vi "ARM2 Reset parameters.vi"(0 "ARM2 Y-Galvo Offset":dbl, 1 "ARM2 Obejective Offset":dbl(slide) scale=0.0..10.0, 5 "ARM2 Z-Galvo Offset":dbl, 7 "ARM1 Z-Galvo Offset":dbl(slide) scale=0.0..10.0, 11 "ARM1 Obejective Offset":dbl(slide) scale=0.0..10.0, 12 "ARM1 Y-Galvo Offset":dbl(slide) scale=0.0..10.0) -> (4 "DAQ 2":waveform(dbl)[](array[waveform]), 15 "DAQ1":waveform(dbl)[](array[waveform]))   [LabVIEW 2016]
uses:
  <vilib>/measure/NI_MABase.lvlib
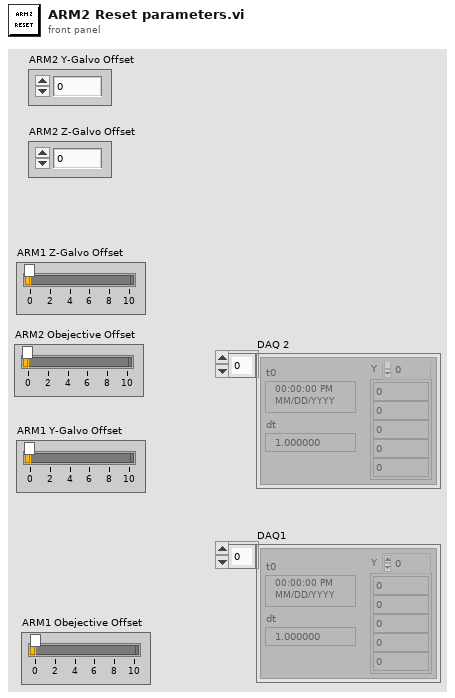
[diagram p1: front panel]
types:
  T1 = enum16{"Sine Wave", "Triangle Wave", "Square Wave", "Sawtooth Wave"}
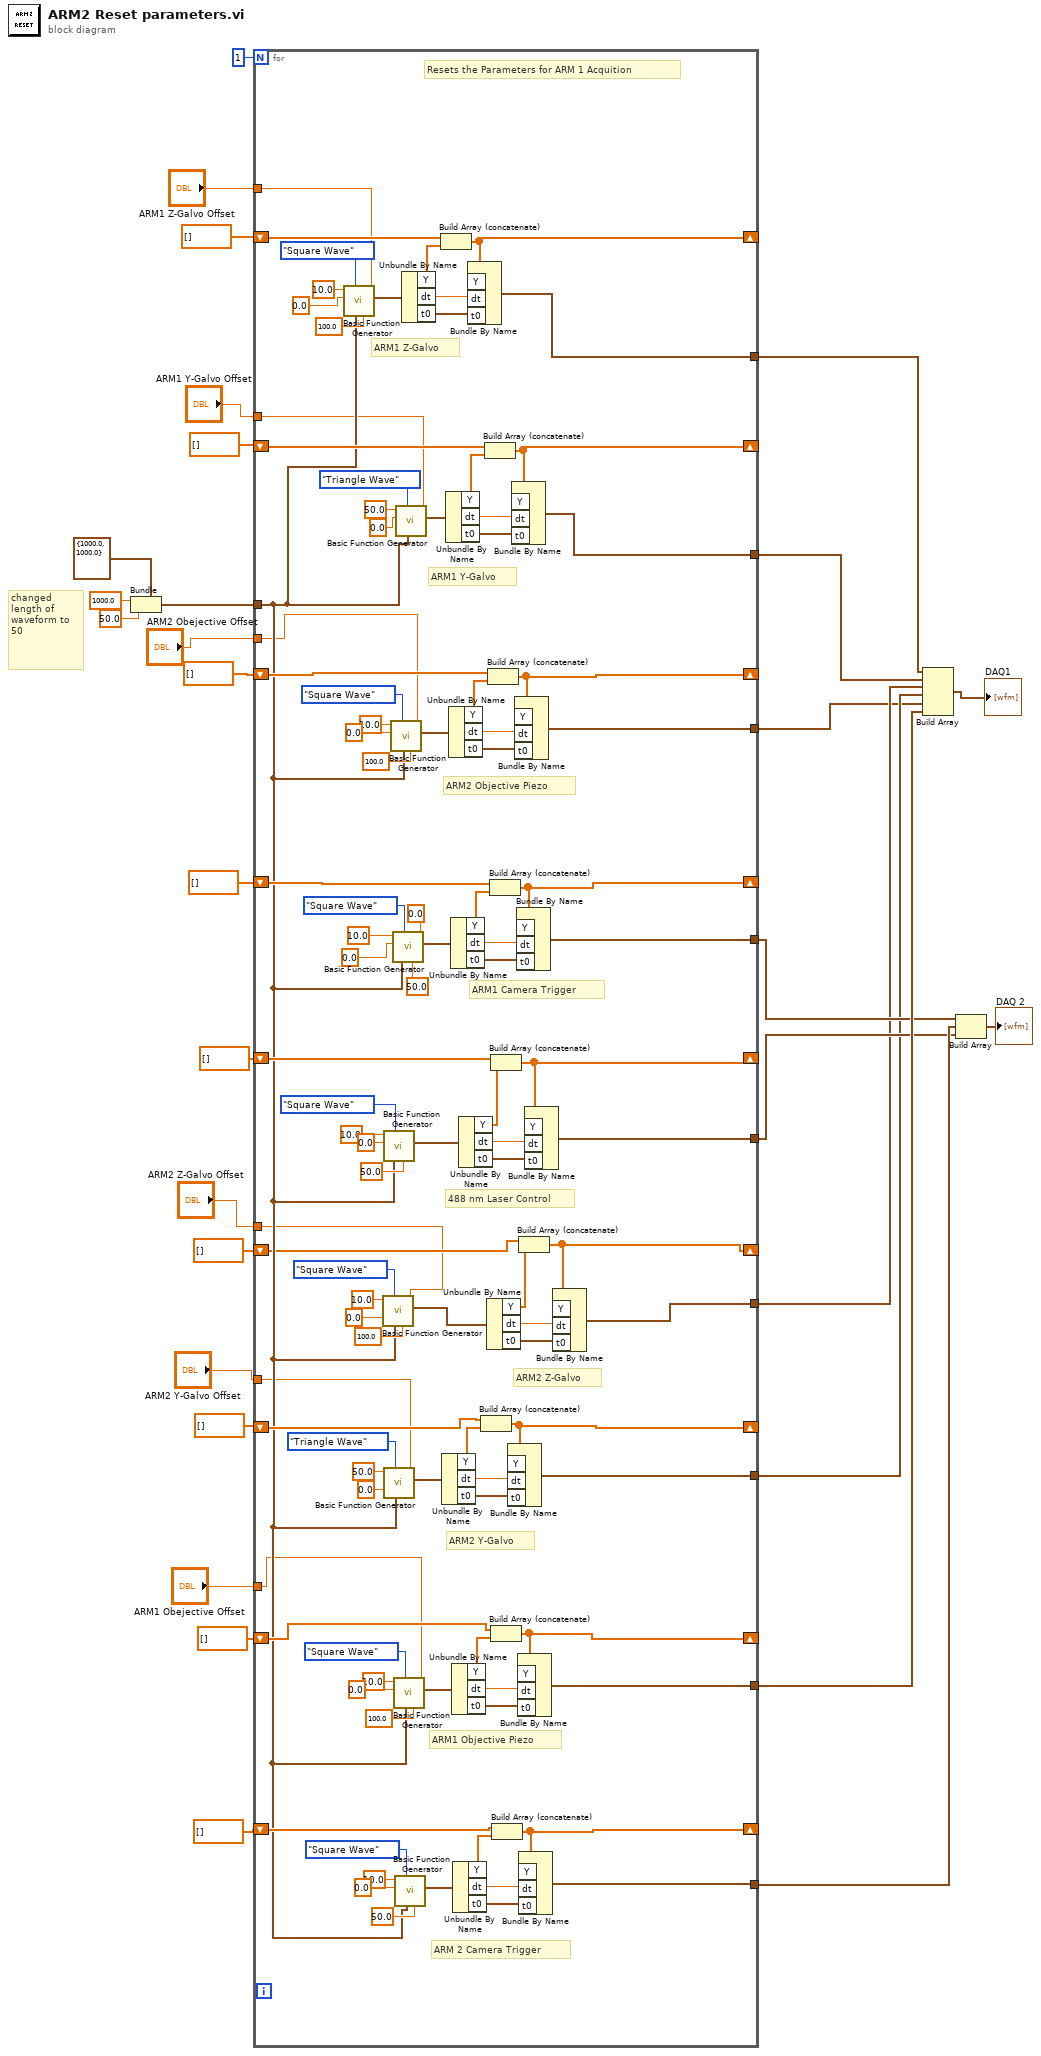
[diagram p0: block diagram]
diagram:
  # "changed length of waveform to 50"
  n1 = Bundle(cluster=cluster{"Fs":dbl, "#s":dbl} {"Fs"=1000.0, "#s"=1000.0} ("sampling info"), "Fs"=1000.0, "#s"=50.0) -> (w28:cluster{"Fs":dbl, "#s":dbl})
  n2 = for {
    N: 1 -> [_]
    shift-right: [w128] -> _
    shift-left: dbl[] [] ("appended array") -> [w129]
    tunnel: [w127] -> w22
    shift-right: [w121] -> _
    shift-left: dbl[] [] ("appended array") -> [w122]
    tunnel: [w120] -> w13
    tunnel: w28 -> [w56]
    shift-right: [w99] -> _
    shift-left: dbl[] [] ("appended array") -> [w100]
    tunnel: [w98] -> w1
    shift-right: [w96] -> _
    shift-left: dbl[] [] ("appended array") -> [w97]
    tunnel: [w95] -> w12
    tunnel: "ARM1 Z-Galvo Offset" -> [w38]
    tunnel: "ARM1 Y-Galvo Offset" -> [w37]
    tunnel: "ARM2 Obejective Offset" -> [w36]
    tunnel: [w44] -> w3
    tunnel: [w74] -> w2
    tunnel: [w73] -> w21
    tunnel: [w72] -> w20
    shift-right: [w70] -> _
    shift-left: dbl[] [] ("appended array") -> [w71]
    shift-right: [w68] -> _
    shift-left: dbl[] [] ("appended array") -> [w69]
    shift-right: [w66] -> _
    shift-left: dbl[] [] ("appended array") -> [w67]
    tunnel: "ARM1 Obejective Offset" -> [w33]
    shift-right: [w58] -> _
    shift-left: dbl[] [] ("appended array") -> [w62]
    tunnel: [w63] -> w8
    tunnel: "ARM2 Y-Galvo Offset" -> [w34]
    shift-right: [w46] -> _
    shift-left: dbl[] [] ("appended array") -> [w45]
    tunnel: "ARM2 Z-Galvo Offset" -> [w35]
    # "ARM2 Z-Galvo"
    # "Resets the Parameters for ARM 1 Acquition"
    # "ARM 2 Camera Trigger"
    # "ARM1 Objective Piezo"
    # "ARM2 Y-Galvo"
    # "488 nm Laser Control"
    # "ARM1 Camera Trigger"
    # "ARM2 Objective Piezo"
    # "ARM1 Y-Galvo"
    # "ARM1 Z-Galvo"
    n3 = call <vilib>:"Basic Function Generator.vi"("offset"=w38, "square wave duty cycle (%)"=100.0, "sampling info"=w56, "signal type"=T1."Square Wave", "amplitude"=0.0, "frequency"=10.0) -> ("signal out"=w130:waveform(dbl))  [unwired: 3 in, 2 out]
    n4 = call <vilib>:"Basic Function Generator.vi"("offset"=w35, "square wave duty cycle (%)"=100.0, "sampling info"=w56, "signal type"=T1."Square Wave", "amplitude"=0.0, "frequency"=10.0) -> ("signal out"=w47:waveform(dbl))  [unwired: 3 in, 2 out]
    n5 = call <vilib>:"Basic Function Generator.vi"("square wave duty cycle (%)"=50.0, "sampling info"=w56, "signal type"=T1."Square Wave", "amplitude"=0.0, "frequency"=10.0) -> ("signal out"=w64:waveform(dbl))  [unwired: 4 in, 2 out]
    n6 = call <vilib>:"Basic Function Generator.vi"("offset"=w34, "sampling info"=w56, "signal type"=T1."Triangle Wave", "amplitude"=0.0, "frequency"=50.0) -> ("signal out"=w91:waveform(dbl))  [unwired: 4 in, 2 out]
    n7 = call <vilib>:"Basic Function Generator.vi"("offset"=w36, "square wave duty cycle (%)"=100.0, "sampling info"=w56, "signal type"=T1."Square Wave", "amplitude"=0.0, "frequency"=10.0) -> ("signal out"=w113:waveform(dbl))  [unwired: 3 in, 2 out]
    n8 = call <vilib>:"Basic Function Generator.vi"("offset"=0.0, "square wave duty cycle (%)"=50.0, "sampling info"=w56, "signal type"=T1."Square Wave", "amplitude"=0.0, "frequency"=10.0) -> ("signal out"=w107:waveform(dbl))  [unwired: 3 in, 2 out]
    n9 = call <vilib>:"Basic Function Generator.vi"("offset"=w33, "square wave duty cycle (%)"=100.0, "sampling info"=w56, "signal type"=T1."Square Wave", "amplitude"=0.0, "frequency"=10.0) -> ("signal out"=w84:waveform(dbl))  [unwired: 3 in, 2 out]
    n10 = call <vilib>:"Basic Function Generator.vi"("square wave duty cycle (%)"=50.0, "sampling info"=w56, "signal type"=T1."Square Wave", "amplitude"=0.0, "frequency"=10.0) -> ("signal out"=w77:waveform(dbl))  [unwired: 4 in, 2 out]
    n11 = call <vilib>:"Basic Function Generator.vi"("offset"=w37, "sampling info"=w56, "signal type"=T1."Triangle Wave", "amplitude"=0.0, "frequency"=50.0) -> ("signal out"=w123:waveform(dbl))  [unwired: 4 in, 2 out]
    n12 = Unbundle By Name(w130) -> ("Y"=w131:dbl[], "dt"=w118:dbl, "t0"=w119:timestamp)
    n13 = Build Array (concatenate)(w129, w131) -> (w128:dbl[])
    n14 = Unbundle By Name(w91) -> ("Y"=w92:dbl[], "dt"=w89:dbl, "t0"=w90:timestamp)
    n15 = Unbundle By Name(w123) -> ("Y"=w124:dbl[], "dt"=w125:dbl, "t0"=w126:timestamp)
    n16 = Unbundle By Name(w113) -> ("Y"=w114:dbl[], "dt"=w111:dbl, "t0"=w112:timestamp)
    n17 = Unbundle By Name(w107) -> ("Y"=w108:dbl[], "dt"=w105:dbl, "t0"=w106:timestamp)
    n18 = Unbundle By Name(w84) -> ("Y"=w85:dbl[], "dt"=w82:dbl, "t0"=w83:timestamp)
    n19 = Unbundle By Name(w77) -> ("Y"=w78:dbl[], "dt"=w75:dbl, "t0"=w76:timestamp)
    n20 = Unbundle By Name(w64) -> ("Y"=w61:dbl[], "dt"=w60:dbl, "t0"=w59:timestamp)
    n21 = Bundle By Name("Y"=w128, "dt"=w118, "t0"=w119) -> (w127:waveform(dbl))  [unwired: 1 in]
    n22 = Build Array (concatenate)(w71, w92) -> (w70:dbl[])
    n23 = Build Array (concatenate)(w122, w124) -> (w121:dbl[])
    n24 = Unbundle By Name(w47) -> ("Y"=w50:dbl[], "dt"=w49:dbl, "t0"=w48:timestamp)
    n25 = Build Array (concatenate)(w100, w114) -> (w99:dbl[])
    n26 = Build Array (concatenate)(w97, w108) -> (w96:dbl[])
    n27 = Build Array (concatenate)(w62, w61) -> (w58:dbl[])
    n28 = Build Array (concatenate)(w69, w85) -> (w68:dbl[])
    n29 = Build Array (concatenate)(w67, w78) -> (w66:dbl[])
    n30 = Bundle By Name("Y"=w70, "dt"=w89, "t0"=w90) -> (w74:waveform(dbl))  [unwired: 1 in]
    n31 = Bundle By Name("Y"=w121, "dt"=w125, "t0"=w126) -> (w120:waveform(dbl))  [unwired: 1 in]
    n32 = Bundle By Name("Y"=w99, "dt"=w111, "t0"=w112) -> (w98:waveform(dbl))  [unwired: 1 in]
    n33 = Bundle By Name("Y"=w96, "dt"=w105, "t0"=w106) -> (w95:waveform(dbl))  [unwired: 1 in]
    n34 = Bundle By Name("Y"=w68, "dt"=w82, "t0"=w83) -> (w73:waveform(dbl))  [unwired: 1 in]
    n35 = Build Array (concatenate)(w45, w50) -> (w46:dbl[])
    n36 = Bundle By Name("Y"=w66, "dt"=w75, "t0"=w76) -> (w72:waveform(dbl))  [unwired: 1 in]
    n37 = Bundle By Name("Y"=w58, "dt"=w60, "t0"=w59) -> (w63:waveform(dbl))  [unwired: 1 in]
    n38 = Bundle By Name("Y"=w46, "dt"=w49, "t0"=w48) -> (w44:waveform(dbl))  [unwired: 1 in]
  }
  n39 = Build Array(w22, w13, w3, w2, w1, w21) -> (→"DAQ1":waveform(dbl)[])
  n40 = Build Array(w12, w20, w8) -> (→"DAQ 2":waveform(dbl)[])
